vi "Check if Exe.vi"() -> (0 "Executable Application?":bool)   [LabVIEW 2020]
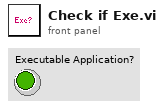
[diagram p1: front panel]
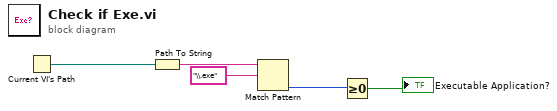
[diagram p0: block diagram]
diagram:
  n1 = Current VI's Path() -> (path=w3:path)
  n2 = Path To String(path=w3) -> (string=w2:string)
  n3 = Match Pattern(string=w2, regular expression="\\.exe") -> (offset past match=w4:i32)  [unwired: 1 in, 3 out]
  n4 = Greater Or Equal To 0?(x=w4) -> (x >= 0?=→"Executable Application?":bool)
